vi "Volts_to_temperature_(SubVI).vi"(4 "Resistance":i32, 7 "error in":errorcluster, 16 "koeff. cluster":T1 {"R0" format="%#_18g"; "k7" format="%#_18g"; "k6" format="%#_18g"; "k5" format="%#_18g"; "k4" format="%#_18g"; "k3" format="%#_18g"; "k2" format="%#_18g"; "k1" format="%#_18g"}) -> (9 "s? color":u32, 10 "Vin < 0?":bool, 20 "T solvation":dbl, 21 "meas_voltage":dbl, 27 "error out":errorcluster)   [LabVIEW 2015]
uses:
  <vilib>/express/express arith-compare/Formula/XNode/ExpressFormulaBlockNode.xnode
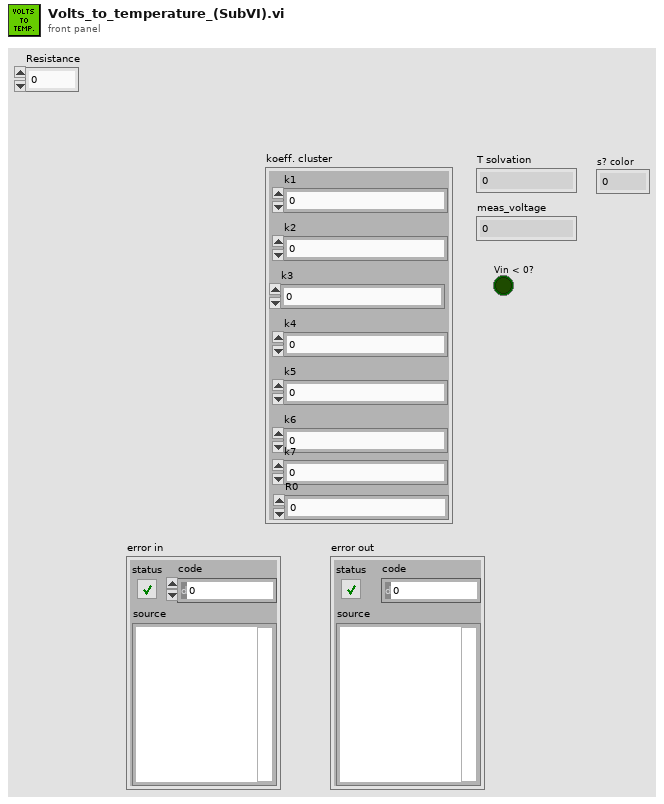
[diagram p1: front panel]
types:
  T1 = cluster{"k1":ext, "k2":ext, "k3":ext, "k4":ext, "k5":ext, "k6":ext, "k7":ext, "R0":ext}
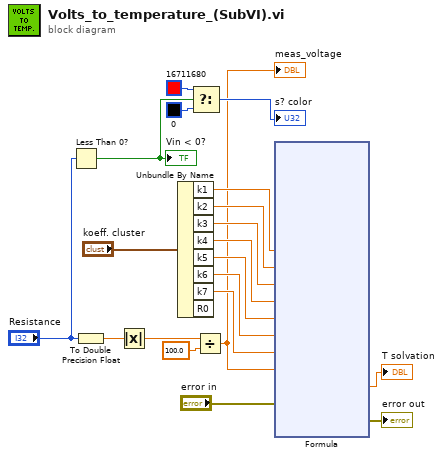
[diagram p0: block diagram]
diagram:
  n1 = Less Than 0?(x="Resistance") -> (x < 0?=w18:bool)
  "Vin < 0?" <- w18
  n2 = To Double Precision Float(number="Resistance") -> (double precision float=w16:dbl)
  n3 = Absolute Value(x=w16) -> (abs(x)=w14:dbl)
  n4 = Unbundle By Name("koeff. cluster") -> ("k1"=w11:ext, "k2"=w10:ext, "k3"=w9:ext, "k4"=w8:ext, "k5"=w7:ext, "k6"=w6:ext, "k7"=w5:ext)  [unwired: 1 out]
  n5 = Select(t=u32 16711680, s=w18, f=u32 0) -> (s? t:f=→"s? color":u32)
  n6 = Divide(x=w14, y=100.0) -> (x/y=w1:dbl)
  "meas_voltage" <- w1
  n7 = xnode "Formula"("k1"=w11, "k2"=w10, "k3"=w9, "k4"=w8, "k5"=w7, "k6"=w6, "k7"=w5, "Rin"=w1, "error in (no error)"="error in") -> ("Result"=→"T solvation":ext, "error out"=→"error out":errorcluster)
